vi "Save_Destination_Type.vi"(8 "error in (no error)":errorcluster, 9 "index":string, 10 "buildObject":T1, 11 "Dest_User_MSIPath in":refnum<class "Dest_User_MSIPath.lvclass">) -> (0 "error out":errorcluster, 1 "index out":string, 2 "buildObject out":T1, 3 "Dest_User_MSIPath out":refnum<class "Dest_User_MSIPath.lvclass">)   [LabVIEW 2020, in "Dest_User_MSIPath.lvclass"]
uses:
  <vilib>/AppBuilder/IB_Classes/Dest_User_MSIPath/Dest_User_MSIPath.lvclass
  <vilib>/AppBuilder/IB_Classes/Dest_User_MSIPath/Dest_User_MSIPath.lvclass/Dest_User_MSIPath.ctl
  <resource>/Framework/Providers/API/ItemRef.ctl
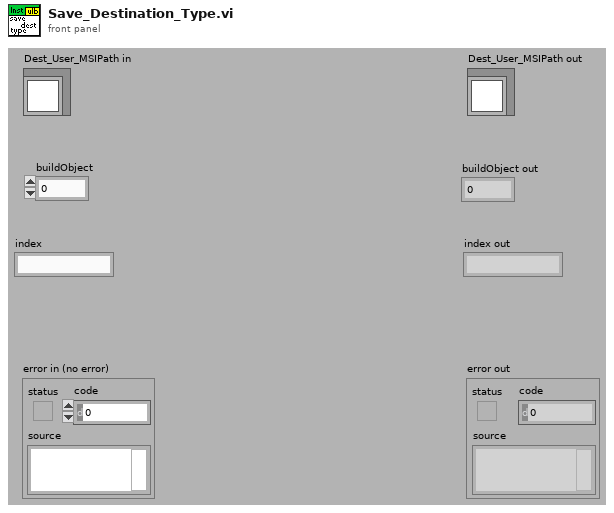
[diagram p1: front panel]
types:
  T1 = typedef "ItemRef.ctl" = u64
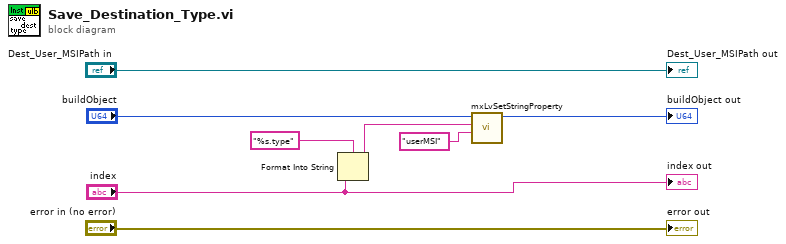
[diagram p0: block diagram]
diagram:
  n1 = Format Into String(format string="%s.type", "index") -> (resulting string=w7:string)  [unwired: 2 in, 1 out]
  n2 = call <resource>:"mxLvSetStringProperty.vi"("Value (\"\")"="userMSI" ("Value (\"\")"), "Tag"=w7, "Item"="buildObject") -> ("Item"=→"buildObject out":T1)  [unwired: 7 in, 1 out]
  "error out" <- "error in (no error)"
  "Dest_User_MSIPath out" <- "Dest_User_MSIPath in"
  "index out" <- "index"
